vi "python_node_example_2023_Q1.vi"() -> ()   [LabVIEW 2023]
panel:
  out "appended path":path
  out "return_tuple":cluster{i32, i32, bool[]}
  out "return_dict":T1
  out "return_tuple_list":cluster{i32, i32, bool[]}[](array[cluster])
  out "return_list":bool[](array[boolean])
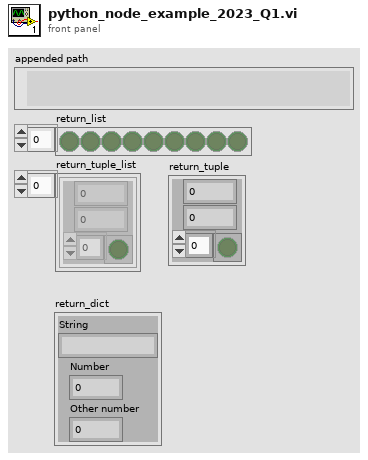
[diagram p1: front panel]
types:
  T1 = cluster{"String":string, "Number":i32, "Other number":i32}
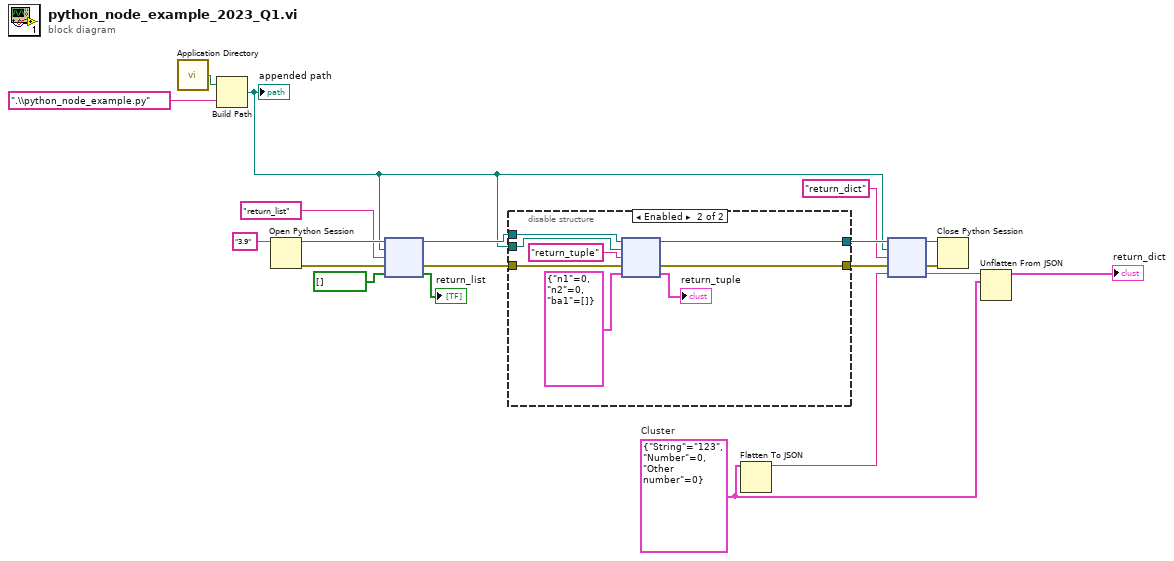
[diagram p0: block diagram]
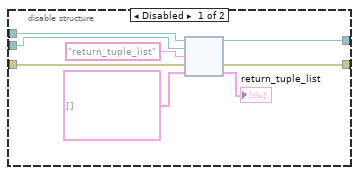
[diagram p2: hidden frame]
diagram:
  w4 = T1 {"String"="123", "Number"=0, "Other number"=0}  # Cluster
  n1 = call <vilib>:"Application Directory.vi"() -> ("Application Directory"=w20:path)
  n2 = Build Path(base path=w20, name or relative path=".\\python_node_example.py") -> (appended path=w1:path)
  "appended path" <- w1
  n3 = Open Python Session(python version="3.9" ("Python version")) -> (session out=w18:refnum<k35>, error out=w17:errorcluster)  [unwired: 2 in]
  n4 = node(w18, w1, "return_list" ("function name"), w17, bool[] []) -> (w12:refnum<k35>, w11:errorcluster, →"return_list":bool[])  [unwired: 2 out]
  n5 = disable-structure shown="Enabled" {
    disable-tunnel: w12 -> [w27 w35]
    disable-tunnel: w11 -> [w26 w34]
    disable-tunnel: [w25 w33] -> w10
    disable-tunnel: [w24 w32] -> w9
    disable-tunnel: w1 -> [w21 w31]
    frame Disabled {
      n6 = node(w27, w21, "return_tuple_list" ("function name"), w26, cluster{i32, i32, bool[]}[] []) -> (w25:refnum<k35>, w24:errorcluster, →"return_tuple_list":cluster{i32, i32, bool[]}[])  [unwired: 2 out]
    }
    frame Enabled {
      n7 = node(w35, w31, "return_tuple" ("function name"), w34, cluster{"n1":i32, "n2":i32, "ba1":bool[]} {"n1"=0, "n2"=0, "ba1"=[]} ("Cluster")) -> (w33:refnum<k35>, w32:errorcluster, →"return_tuple":cluster{"n1":i32, "n2":i32, "ba1":bool[]})  [unwired: 2 out]
    }
  }
  n8 = Flatten To JSON(anything=w4) -> (JSON string=w6:string)  [unwired: 2 in, 1 out]
  n9 = node(w10, w1, "return_dict" ("function name"), w9, w6) -> (w14:refnum<k35>, w13:errorcluster, w5:string)  [unwired: 2 out]
  n10 = Close Python Session(session in=w14, error in=w13) -> ()  [unwired: 1 out]
  n11 = Unflatten From JSON(JSON string=w5, type and defaults=w4) -> (value=→"return_dict":T1)  [unwired: 5 in, 1 out]
